vi "VCI_Receive.vi"(6 "Len":u32=1, 7 "WaitTime":i32=100, 9 "CANIndex":u32, 10 "DevIndex":u32, 11 "DevType":u32=4) -> (0 "VCI_CAN_OBJ":T1, 1 "CANIndex 2":u32, 2 "DevIndex 2":u32, 3 "DevType 2":u32=4, 4 "Len 2":u32=1, 5 "接收的帧数":u32)   [LabVIEW 2014]
uses:
  ControlCAN.dll
panel:
  out "WaitTime 2":i32=100
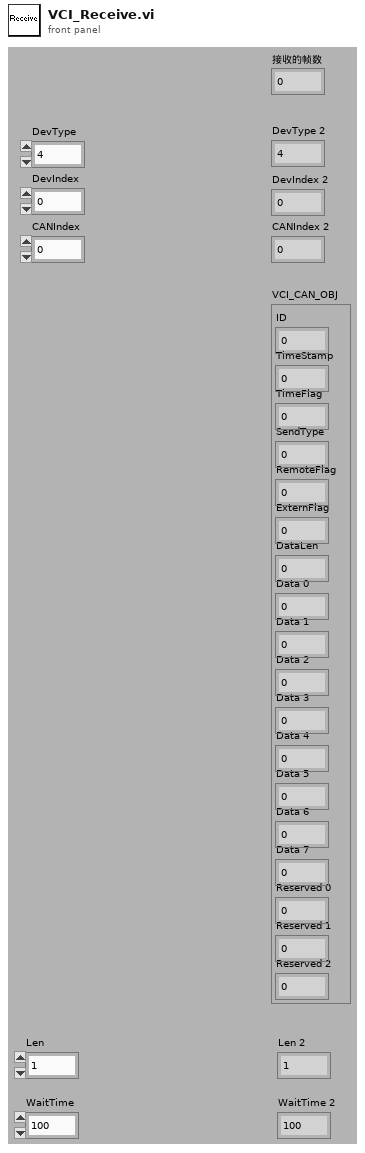
[diagram p1: front panel]
types:
  T1 = cluster{"ID":u32, "TimeStamp":u32, "TimeFlag":u8, "SendType":u8, "RemoteFlag":u8, "ExternFlag":u8, "DataLen":u8, "Data 0":u8, "Data 1":u8, "Data 2":u8, "Data 3":u8, "Data 4":u8, "Data 5":u8, "Data 6":u8, "Data 7":u8, "Reserved 0":u8, "Reserved 1":u8, "Reserved 2":u8}
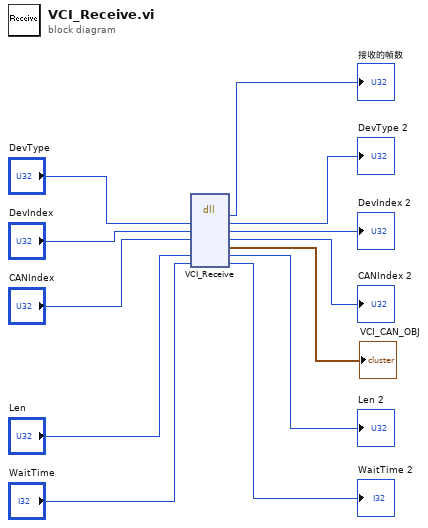
[diagram p0: block diagram]
diagram:
  n1 = dll-call lib="D:/Documents/USBCAN/USBCAN/ControlCAN.dll" fn="VCI_Receive"("DevType"="DevType", "DevIndex"="DevIndex", "CANIndex"="CANIndex", "Len"="Len", "WaitTime"="WaitTime") -> ("帧数"=→"接收的帧数":u32, "DevType"=→"DevType 2":u32, "DevIndex"=→"DevIndex 2":u32, "CANIndex"=→"CANIndex 2":u32, "VCI_CAN_OBJ"=→"VCI_CAN_OBJ":T1, "Len"=→"Len 2":u32, "WaitTime"=→"WaitTime 2":i32)  [unwired: 3 in, 3 out]
